vi "FWUpdate Launch Update UI.vi"(8 "error in (no error)":errorcluster, 10 "API Port (80)":u16=80, 11 "API Server (localhost)":string="localhost") -> (0 "error out":errorcluster)   [LabVIEW 2011]
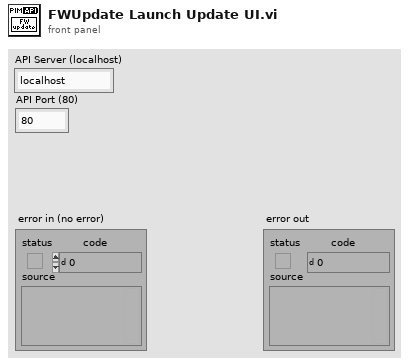
[diagram p1: front panel]
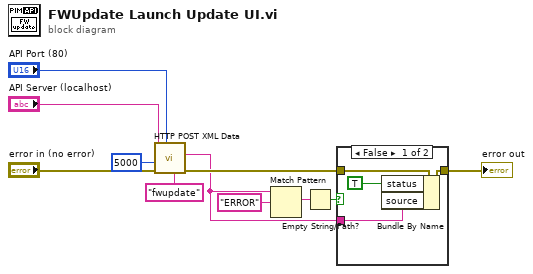
[diagram p0: block diagram]
diagram:
  n1 = call "HTTP POST XML Data.vi"("webService/path (api)"="fwupdate", "port (80)"="API Port (80)", "error in (no error)"="error in (no error)", "Timeout ms (30000)"=5000, "address (localhost)"="API Server (localhost)") -> ("error out"=w8:errorcluster, "XML Response"=w1:string)  [unwired: 3 in, 2 out]
  n2 = Match Pattern(string=w1, regular expression="ERROR") -> (match substring=w7:string)  [unwired: 1 in, 3 out]
  n3 = Empty String/Path?(string/path=w7) -> (empty?=w6:bool)
  n4 = case shown="False" w6 {
    tunnel: w8 -> [w15 w16]
    tunnel: [w13 w16] -> w11
    tunnel: w1 -> [w12 _]
    frame False {
      n5 = Bundle By Name(cluster=w15, "status"=TRUE, "source"=w12) -> (w13:errorcluster)
    }
    frame True {
    }
  }
  "error out" <- w11
